vi "Save Picture Barcode.vi"() -> ()   [LabVIEW 2013]
panel:
  in  "String":string
  in  "Str Refnum":refnum<vi>
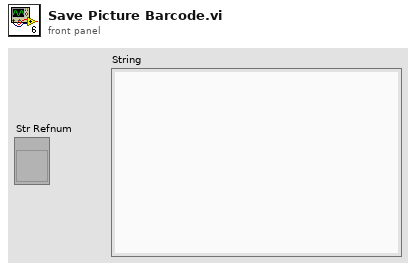
[diagram p1: front panel]
types:
  T1 = typedef "imagedata.ctl" = cluster{"image type":i32, "image depth":i32, "image":u8[], "mask":u8[], "colors":u32[], "Rectangle":cluster{"left":i16, "top":i16, "right":i16, "bottom":i16}}
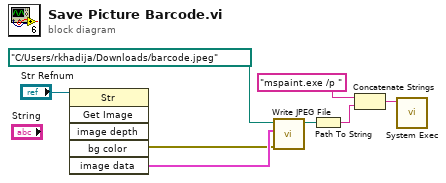
[diagram p0: block diagram]
diagram:
  n1 = invoke on="Invoke Node" class="Str" method="Get Image"(reference="Str Refnum") -> (error out=w6:errorcluster, "image data"=w7:T1)  [unwired: 5 in, 4 out]
  n2 = call <vilib>:"Write JPEG File.vi"("error in (no error)"=w6, "image data"=w7, "path to JPEG file"=path "C:/Users/rkhadija/Downloads/barcode.jpeg") -> ("path"=w4:path)  [unwired: 7 in, 1 out]
  n3 = Path To String(path=w4) -> (string=w3:string)
  n4 = Concatenate Strings("mspaint.exe /p " ("string"), w3) -> (w1:string)
  n5 = call <vilib>:"System Exec.vi"("command line"=w1) -> ()  [unwired: 7 in, 4 out]
